vi "auto adjust sensitivity (no objects).vi"(0 "VISA Resource Name":refnum<visa-resource-name>, 5 "sensitivity":i8, 7 "R value":dbl format="%#_13g", 9 "Input Setting":i32, 11 "error in (no error)":errorcluster) -> (4 "VISA resource name out":refnum<visa-resource-name>, 6 "sensitivity out":i8, 10 "Repeat Measurement?":bool, 15 "error out":errorcluster)   [LabVIEW 2017]
uses:
  Lockin/sr830/SR830.lvlib
panel:
  in  "Post Adjust Wait":dbl[unit]=0.1
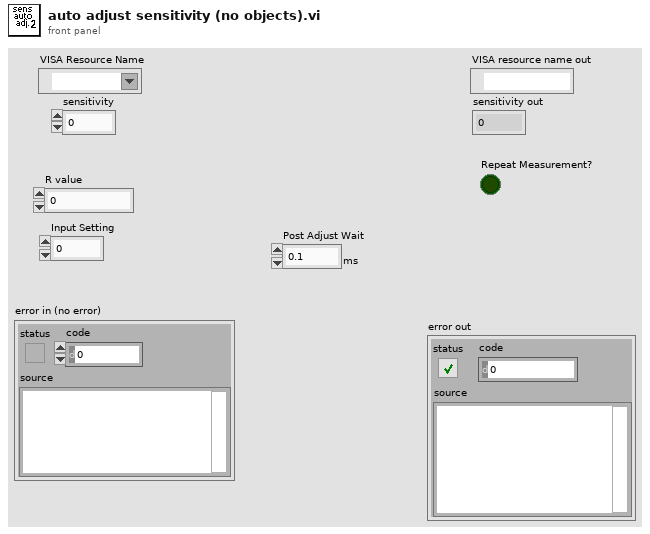
[diagram p1: front panel]
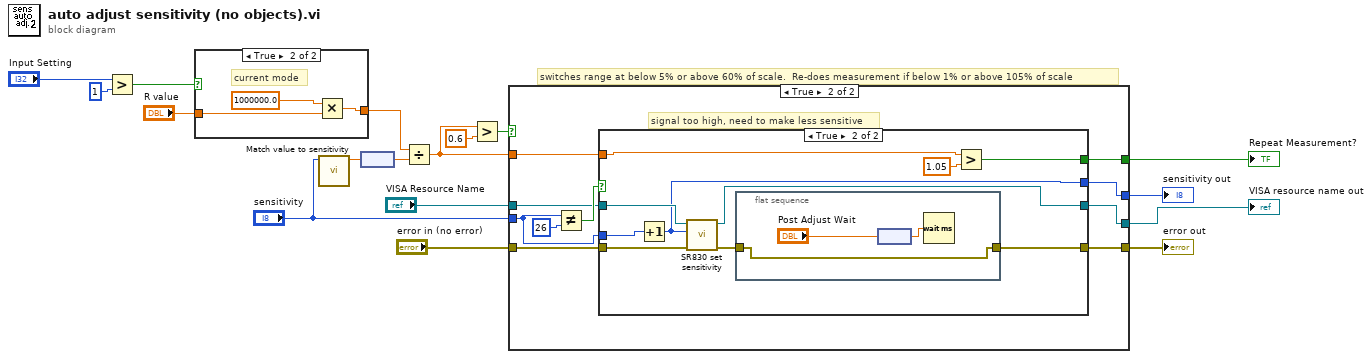
[diagram p0: block diagram]
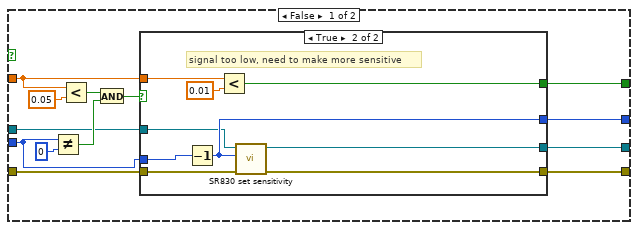
[diagram p2: hidden frame]
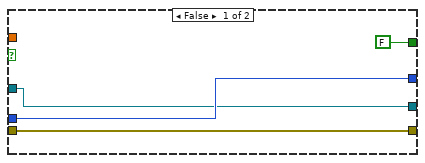
[diagram p3: hidden frame]
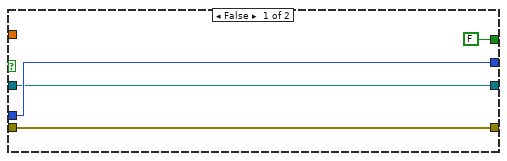
[diagram p4: hidden frame]
diagram:
  # "switches range at below 5% or above 60% of scale.  Re-does measurement if below 1% or above 105% of scale"
  n1 = Greater?(x="Input Setting", y=1) -> (0:w15:bool)
  n2 = case shown="True" w15 {
    tunnel: "R value" -> [w18 w20]
    tunnel: [w18 w19] -> w11
    frame False {
      # "voltage mode"
    }
    frame True {
      # "current mode"
      n3 = Multiply(x=1000000.0, y=w20) -> (x*y=w19:dbl)
    }
  }
  n4 = call "Match value to sensitivity.vi"("integer"="sensitivity") -> ("sensitivity"=w8:dbl[unit])  [unwired: 10 in]
  n5 = node(w8) -> (w9:dbl)
  n6 = Divide(x=w11, y=w9) -> (x/y=w12:dbl)
  n7 = Greater?(x=w12, y=0.6) -> (0:w13:bool)
  n8 = case shown="True" w13 {
    tunnel: "sensitivity" -> [w30 w55]
    tunnel: w12 -> [w24 w54]
    tunnel: "VISA Resource Name" -> [w28 w53]
    tunnel: [w29 w52] -> w1
    tunnel: [w26 w51] -> w6
    tunnel: [w25 w50] -> w7
    tunnel: [w23 w49] -> w2
    tunnel: "error in (no error)" -> [w22 w48]
    frame False {
      n9 = Not Equal?(x=w30, y=0) -> (x != y?=w31:bool)
      n10 = Less?(x=w24, y=0.05) -> (x < y?=w32:bool)
      n11 = And(x=w32, y=w31) -> (x .and. y?=w27:bool)
      n12 = case shown="True" w27 {
        tunnel: w30 -> [w37 w47]
        tunnel: w22 -> [w38 w45]
        tunnel: [w38 w39] -> w29
        tunnel: w28 -> [w35 w44]
        tunnel: [w37 w46] -> w26
        tunnel: [FALSE w41] -> w25
        tunnel: w24 -> [_ w43]
        tunnel: [w35 w40] -> w23
        frame False {
        }
        frame True {
          # "signal too low, need to make more sensitive"
          n13 = Decrement(x=w47) -> (x-1=w46:i8)
          n14 = Less?(x=w43, y=0.01) -> (x < y?=w41:bool)
          n15 = call "SR830 set sensitivity.vi"("error in (no error)"=w45, "Sensitivity"=w46, "VISA resource name"=w44) -> ("error out"=w39:errorcluster, "VISA resource name out"=w40:refnum<visa-resource-name>)  [unwired: 7 in]
        }
      }
    }
    frame True {
      # "signal too high, need to make less sensitive"
      n16 = Not Equal?(x=w55, y=26) -> (x != y?=w56:bool)
      n17 = case shown="True" w56 {
        tunnel: w55 -> [w60 w71]
        tunnel: w54 -> [_ w70]
        tunnel: [FALSE w68] -> w50
        tunnel: w53 -> [w59 w66]
        tunnel: [w58 w67] -> w52
        tunnel: [w60 w65] -> w51
        tunnel: [w59 w64] -> w49
        tunnel: w48 -> [w58 w62]
        frame False {
        }
        frame True {
          n18 = Increment(x=w71) -> (x+1=w65:i8)
          n19 = call "SR830 set sensitivity.vi"("error in (no error)"=w62, "Sensitivity"=w65, "VISA resource name"=w66) -> ("error out"=w63:errorcluster, "VISA resource name out"=w64:refnum<visa-resource-name>)  [unwired: 7 in]
          n20 = flat-sequence {
            tunnel: [w73] -> w67
            tunnel: w63 -> [w73]
            frame #0 {
              n21 = node("Post Adjust Wait") -> (w72:dbl)
              n22 = Wait (ms)(milliseconds to wait=w72) -> ()  [unwired: 1 out]
            }
          }
          n23 = Greater?(x=w70, y=1.05) -> (0:w68:bool)
        }
      }
    }
  }
  "error out" <- w1
  "Repeat Measurement?" <- w7
  "VISA resource name out" <- w2
  "sensitivity out" <- w6
